vi "servo_controller.vi"(6 "pulse length":fxp<+,18,18>, 7 "20 ms counter":fxp<+,18,18>, 9 "trigger state in":fxp<+,1,1>, 11 "counter in":fxp<+,18,18>) -> (1 "trigger state out":fxp<+,1,1>, 3 "counter out":fxp<+,18,18>)   [LabVIEW 2010]
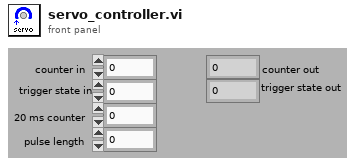
[diagram p1: front panel]
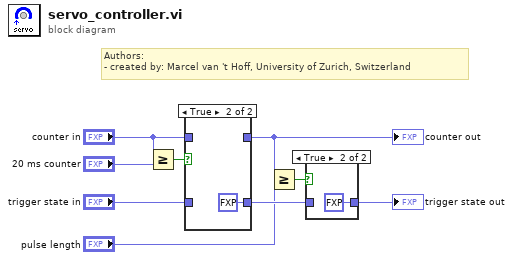
[diagram p0: block diagram]
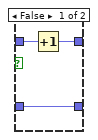
[diagram p3: hidden frame]
diagram:
  # "Authors: \n- created by: Marcel van 't Hoff, University of Zurich, Switzerland"
  n1 = Greater Or Equal?(x="counter in", y="20 ms counter") -> (x >= y?=w3:bool)
  n2 = case shown="True" w3 {
    tunnel: "counter in" -> [w12 _]
    tunnel: [w11 _] -> w7
    tunnel: [w10 fxp<+,1,1> 1.0 ("trigger state in")] -> w9
    tunnel: "trigger state in" -> [w10 _]
    frame False {
      n3 = Increment(x=w12) -> (x+1=w11:fxp<+,18,18>)
    }
    frame True {
    }
  }
  "counter out" <- w7
  n4 = Greater Or Equal?(x=w7, y="pulse length") -> (x >= y?=w6:bool)
  n5 = case shown="True" w6 {
    tunnel: [w14 fxp<+,1,1> 0.0 ("trigger state in")] -> w1
    tunnel: w9 -> [w14 _]
    frame False {
    }
    frame True {
    }
  }
  "trigger state out" <- w1
